vi "Main_Module.vi"(0 "File_hierarchy":string(tree), 11 "Error_In":errorcluster) -> (15 "Error_Out":errorcluster)   [LabVIEW 2023]
uses:
  Controls/Queue_Operation_Select.ctl
  Controls/State_and_Data.ctl
  Controls/Main_Module_Data.ctl
  Classes/Calculator/Calculator.lvclass
  Controls/Object_Data.ctl
  Controls/INI_Operation_Select.ctl
  <vilib>/Utility/miscctls.llb/LVMapReplaceAction.ctl
  Controls/Object_and_instance.ctl
  Drivers/QD_Main.vi
  Drivers/QD_Calci.vi
panel:
  in  "Load":bool
  in  "Save":bool
  in  "Delete":bool
  in  "Add":bool
  in  "Math_Functions":T1(ring) caption="Math Functions"
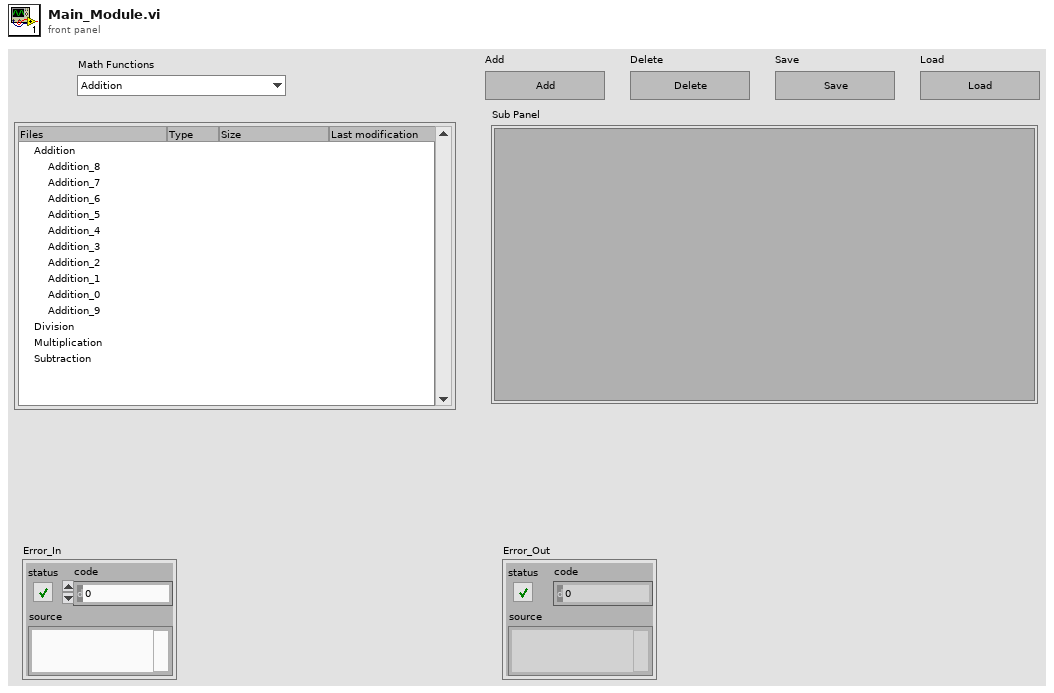
[diagram p1: front panel]
types:
  T1 = enum32{"Addition", "Division", "Multiplication", "Subtraction"}
  T2 = typedef "Queue_Operation_Select.ctl" = enum16{"Obtain_Queue", "Enqueue", "Enqueue_First", "Enqueue_N", "Lossy_Enqueue", "Preview", "Queue_Status", "Dequeue", "Flush", "Release_Queue"}
  T3 = typedef "Main_Module_Data.ctl" = cluster{"File_hierarchy_Reference":refnum<vi>, "Math_Function_Selected":string, "State_and_Data":T4, "Math_Functions":enum16{"Addition", "Division", "Multiplication", "Subtraction"}, "Parent_Class_Path":path, "Calculator.lvclass":refnum<class "Calculator.lvclass">, "Object_Data":T5, "Selected_Tag":string, "Calculator_File_Path":path, "Loaded_VI_Reference":refnum<vi>, "Loaded_Math_Function":string, "Loaded_Tag":string, "Total_Clasees":string[], "INI_File_Path":path}
  T4 = typedef "State_and_Data.ctl" = cluster{"State":string, "Data":variant}
  T5 = typedef "Object_Data.ctl" = map{string, map{string, refnum<class "Calculator.lvclass">}}
  T6 = enum16{"Addition", "Division", "Multiplication", "Subtraction"}
  T7 = typedef "LVMapReplaceAction.ctl" = enum32{"Modify Entry only if found", "Add or Modify Entry", "Delete Entry"}
  T8 = typedef "Object_and_instance.ctl" = cluster{"Object":refnum<class "Calculator.lvclass">, "Insatnce":string}
  T9 = typedef "INI_Operation_Select.ctl" = enum16{"Initialize", "Read", "Read_Key", "Write"}
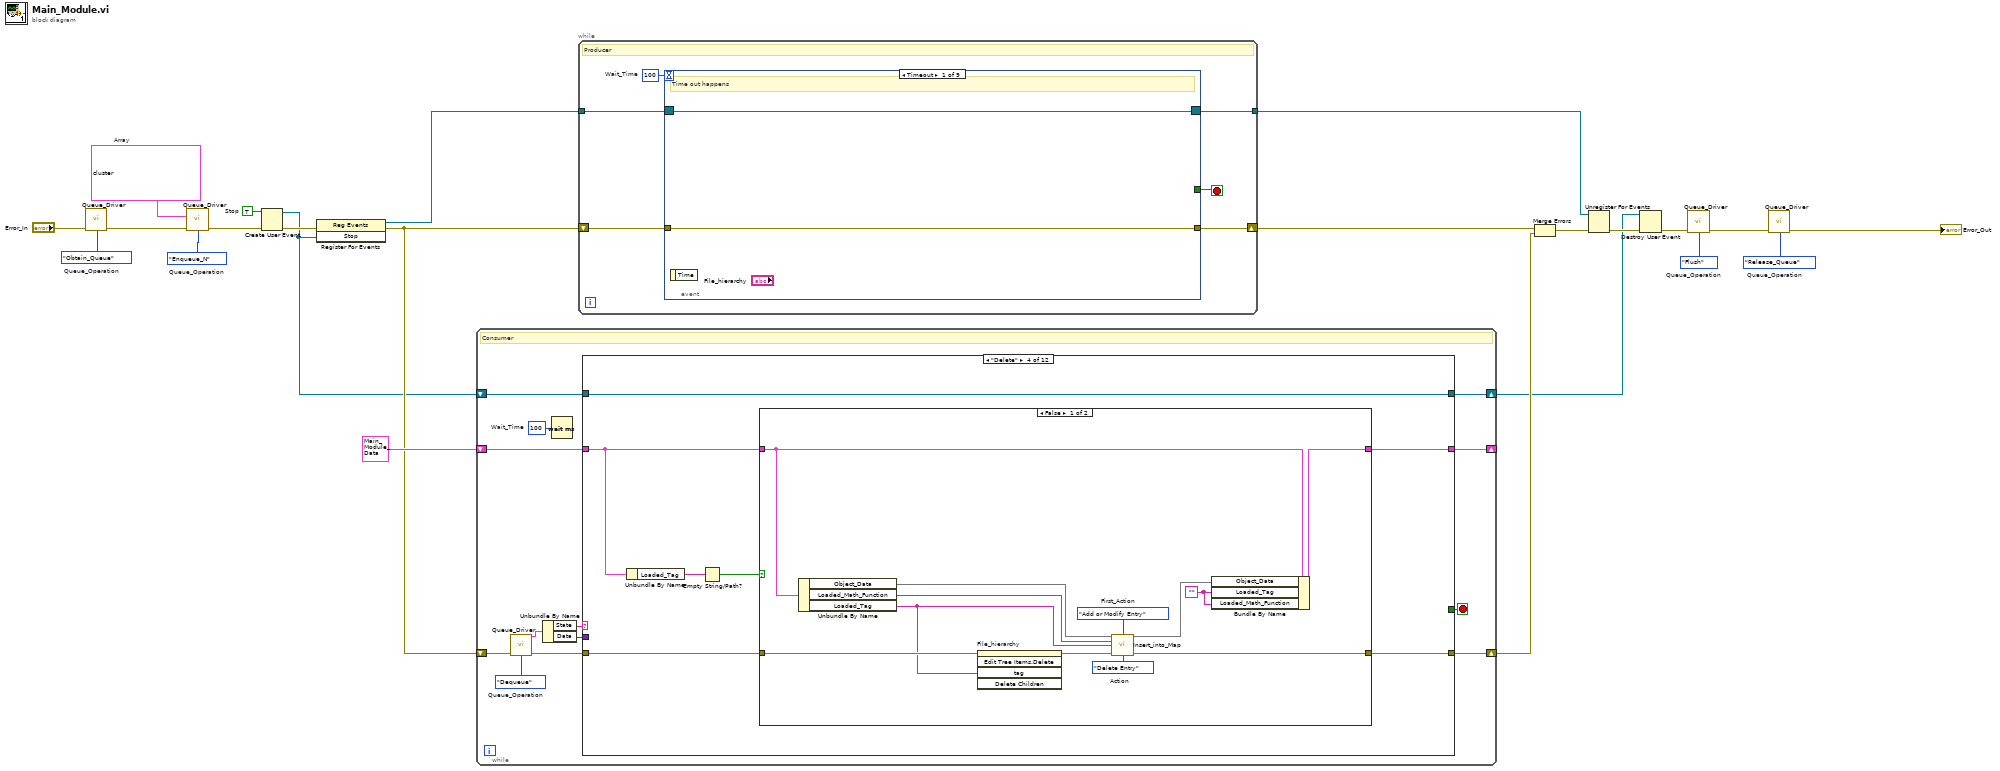
[diagram p0: block diagram]
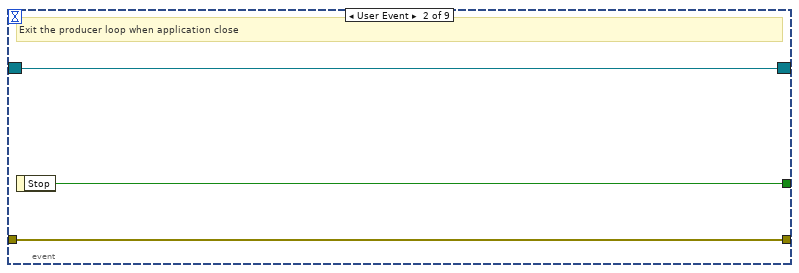
[diagram p2: hidden frame]
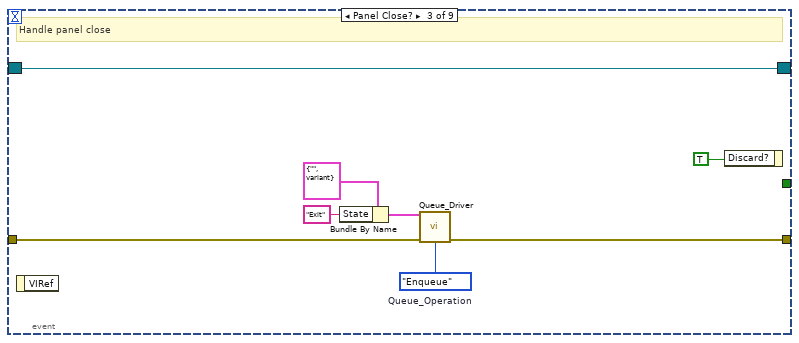
[diagram p3: hidden frame]
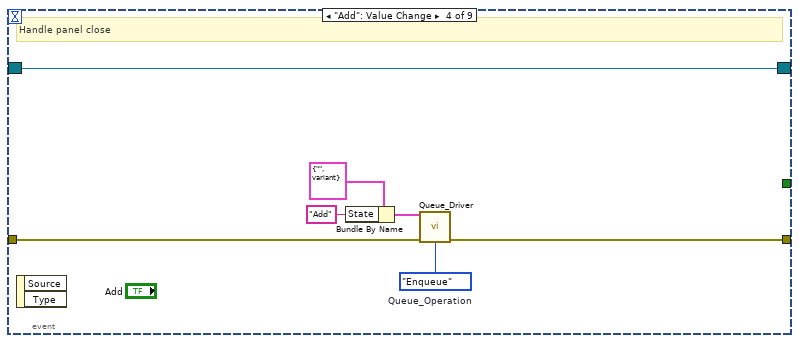
[diagram p4: hidden frame]
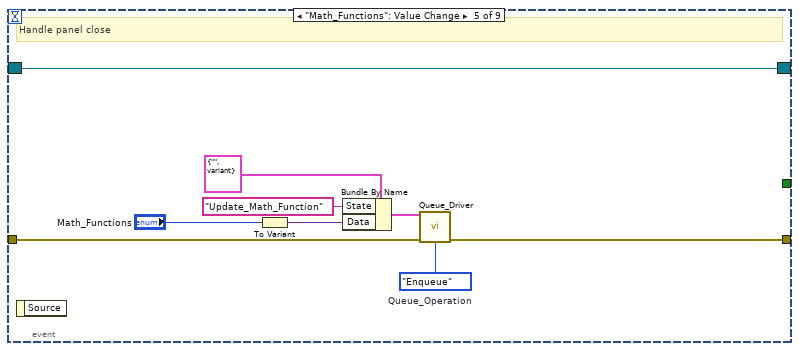
[diagram p5: hidden frame]
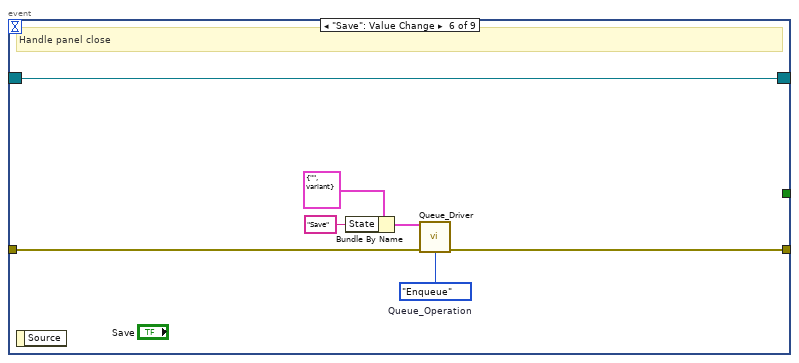
[diagram p6: hidden frame]
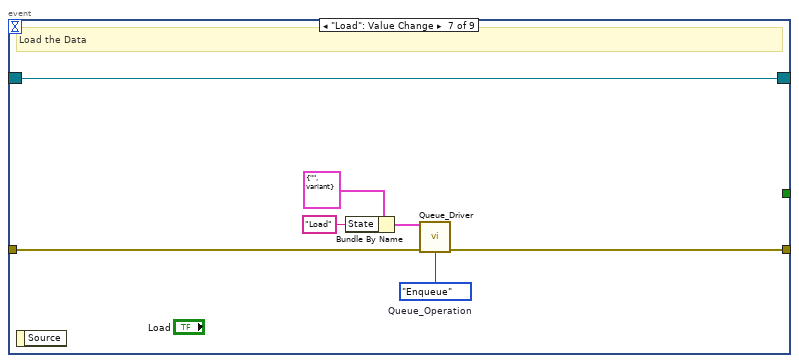
[diagram p7: hidden frame]
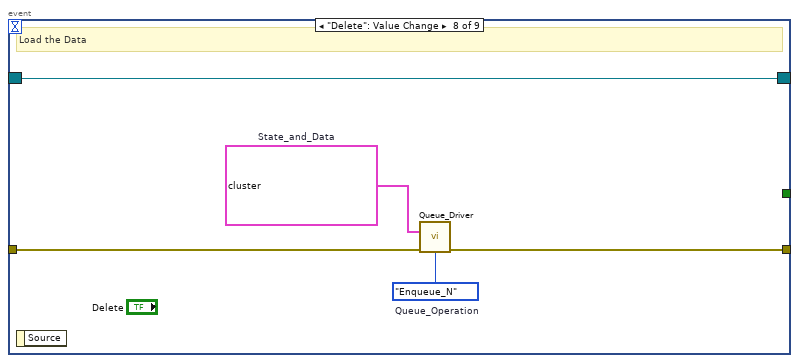
[diagram p8: hidden frame]
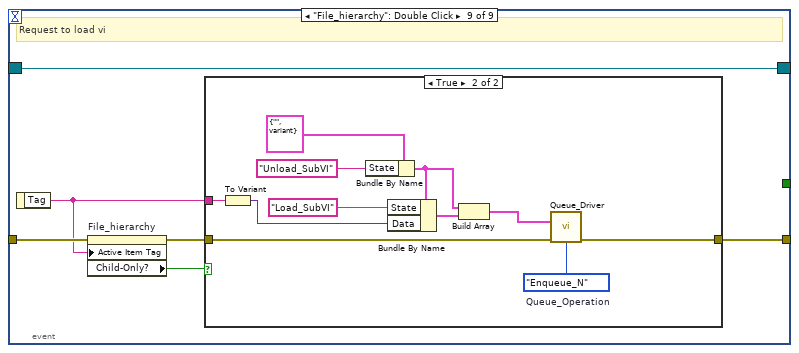
[diagram p9: hidden frame]
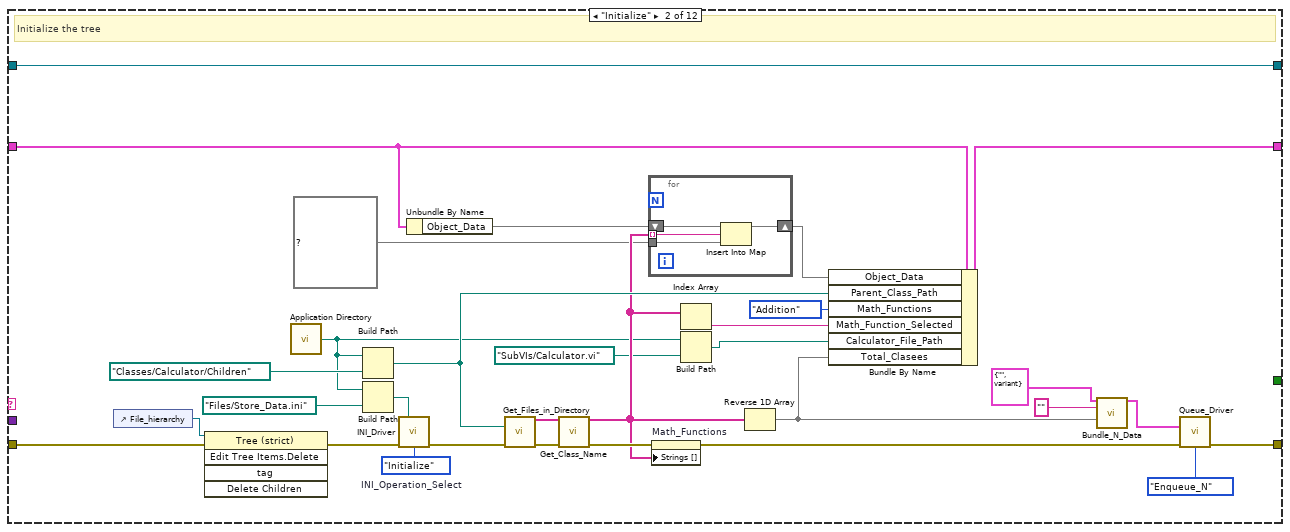
[diagram p12: hidden frame]
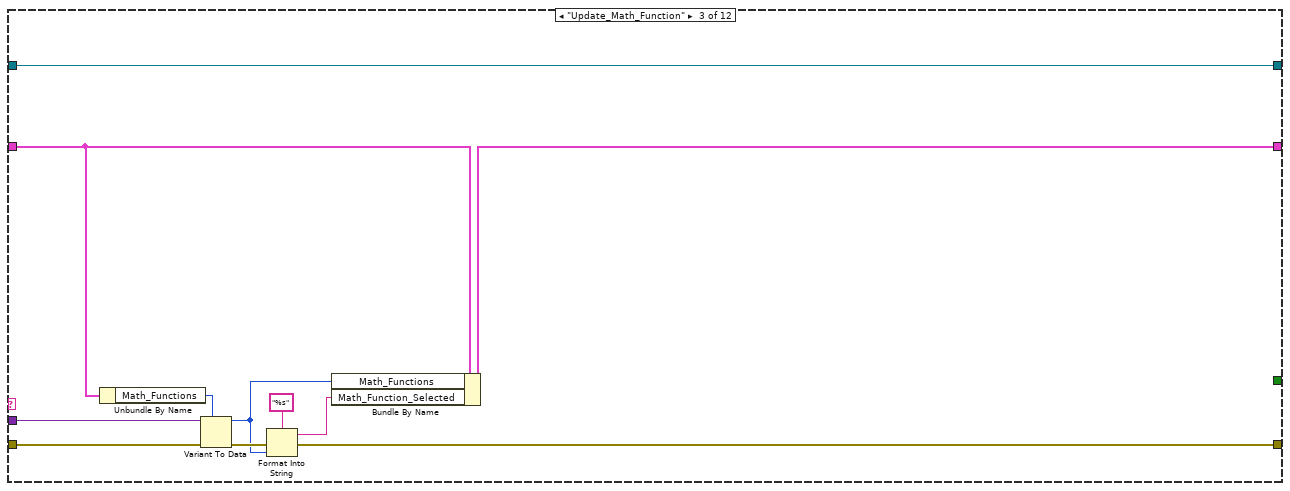
[diagram p13: hidden frame]
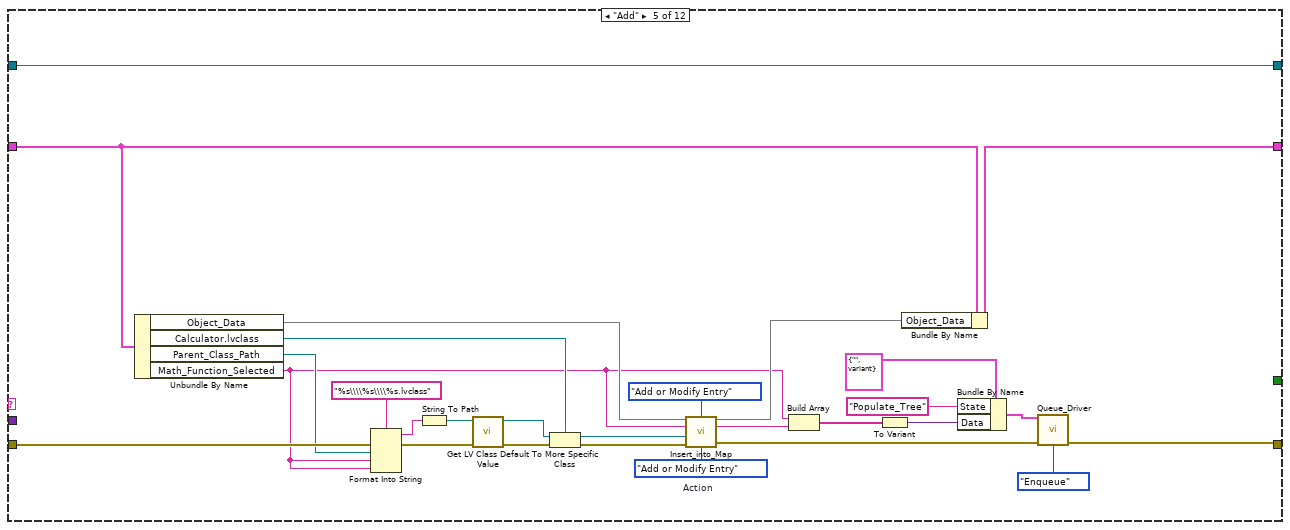
[diagram p15: hidden frame]
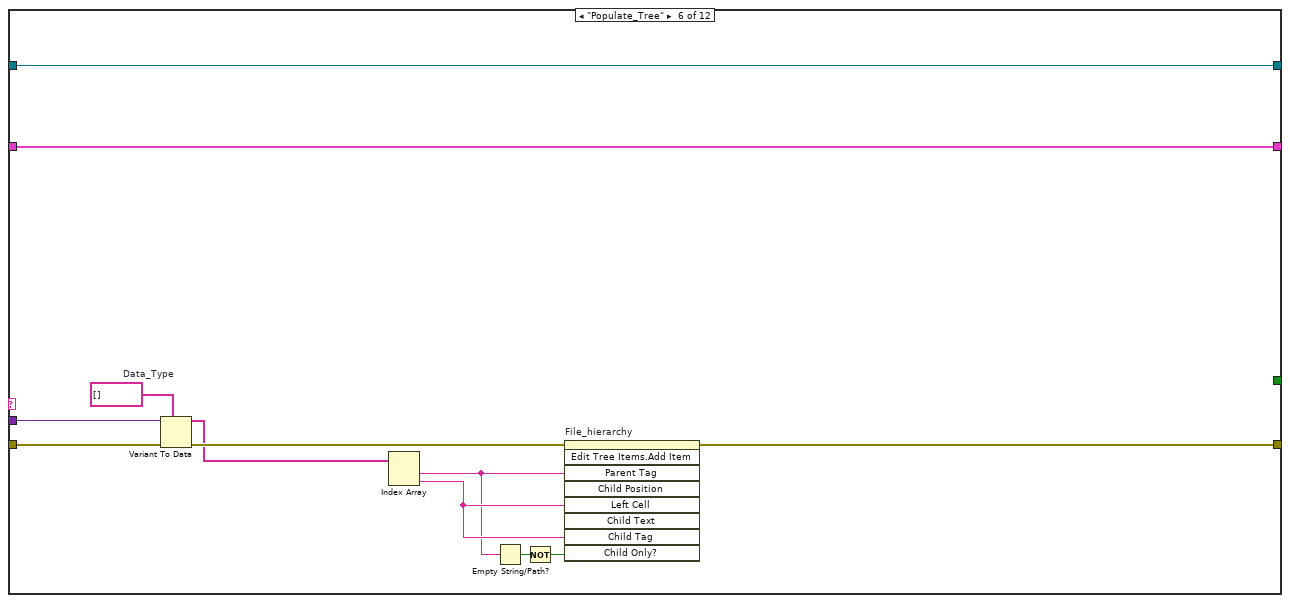
[diagram p16: hidden frame]
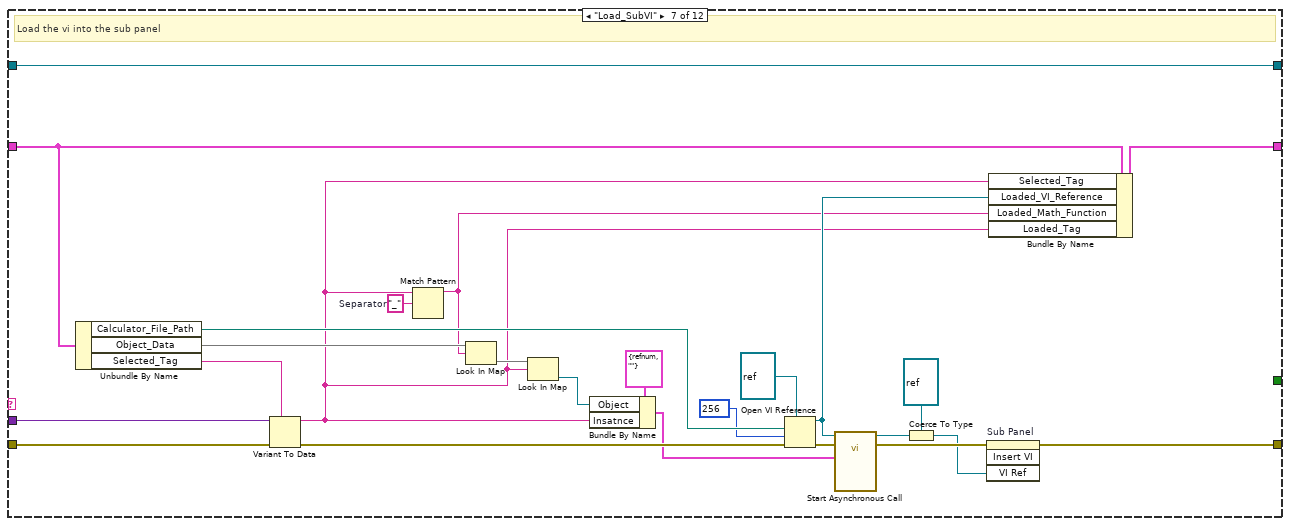
[diagram p17: hidden frame]
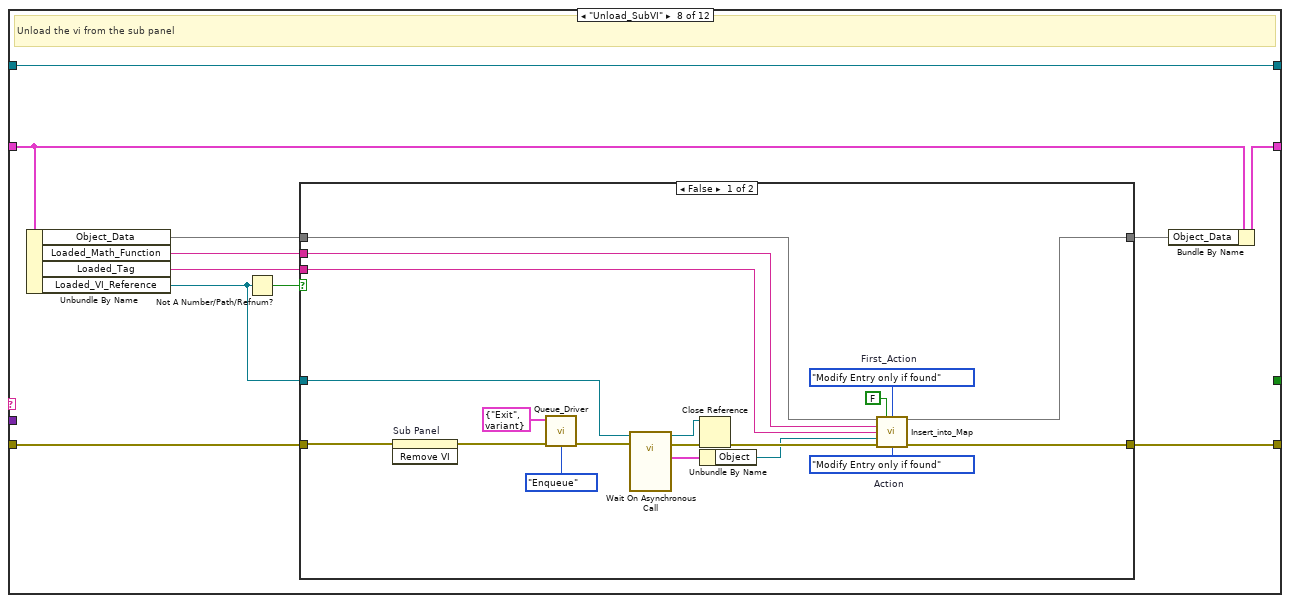
[diagram p18: hidden frame]
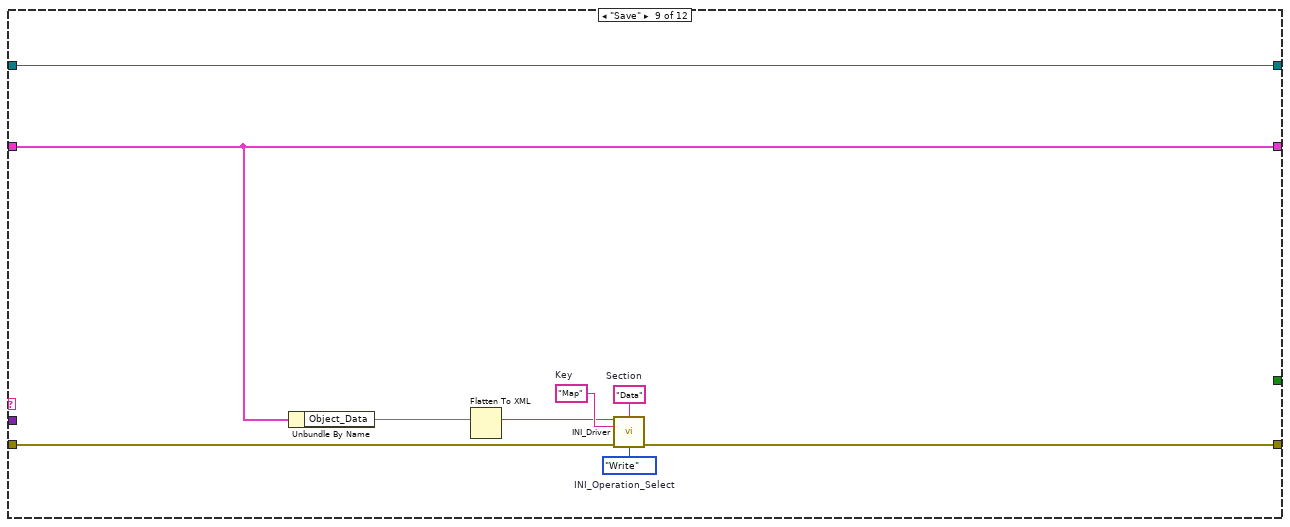
[diagram p20: hidden frame]
diagram:
  w4 = Queue_Operation_Select."Release_Queue"  # Queue_Operation
  w5 = Queue_Operation_Select."Flush"  # Queue_Operation
  w17 = TRUE  # Stop
  w1 = T4[] [{"State"="Initialize", "Data"=variant}, {"State"="Load", "Data"=variant}]  # Array
  w20 = Queue_Operation_Select."Enqueue_N"  # Queue_Operation
  w21 = Queue_Operation_Select."Obtain_Queue"  # Queue_Operation
  n1 = call-poly "Queue_Driver.vi"("Error_In"="Error_In", "Queue_Operation"=w21) -> ("Error_Out"=w22:errorcluster)  [unwired: 11 in, 2 out]
  n2 = call-poly "Queue_Driver.vi"("State_and_Data_N_In"=w1, "Error_In"=w22, "Queue_Operation"=w20) -> ("Error_Out"=w3:errorcluster)  [unwired: 10 in, 2 out]
  n3 = Create User Event(user event datatype=w17, error in=w3) -> (user event=w9:refnum<user-event>, error out=w18:errorcluster)
  n4 = register-events(error in=w18, w9) -> (reference out=w15:refnum<event-registration>, error out=w16:errorcluster)  [unwired: 1 in]
  n5 = while {
    shift-right: [w28] -> w8
    shift-left: w9 -> [w29]
    shift-right: [w27] -> _
    shift-left: T3 {"File_hierarchy_Reference"=refnum, "Math_Function_Selected"="", "State_and_Data"={"State"="", "Data"=variant}, "Math_Functions"=enum."Addition", "Parent_Class_Path"=path "", "Calculator.lvclass"=refnum, "Object_Data"={}, "Selected_Tag"="", "Calculator_File_Path"=path "", "Loaded_VI_Reference"=refnum, "Loaded_Math_Function"="", "Loaded_Tag"="", "Total_Clasees"=[], "INI_File_Path"=path ""} -> [w30]
    shift-right: [w26] -> w13
    shift-left: w16 -> [w36]
    stop <- w25 stop-if-true
    w24 = u32 100  # Wait_Time
    w34 = Queue_Operation_Select."Dequeue"  # Queue_Operation
    # "Consumer"
    n6 = call-poly "Queue_Driver.vi"("Error_In"=w36, "Queue_Operation"=w34) -> ("State_and_Data_Out"=w33:T4, "Error_Out"=w35:errorcluster)  [unwired: 11 in, 1 out]
    n7 = Unbundle By Name(w33) -> ("State"=w32:string, "Data"=w31:variant)
    n8 = Wait (ms)(milliseconds to wait=w24) -> ()  [unwired: 1 out]
    n9 = case shown="\"Delete\"" w32 {
      tunnel: [w39 w61 w78 w90 w116 w143 w169 w179 w210 w213 w248 w258] -> w26
      tunnel: w35 -> [w39 w70 w85 w92 w134 w146 w171 w174 w211 w226 w252 w260]
      tunnel: w31 -> [_ _ w82 _ _ w141 w170 _ _ _ w253 _]
      tunnel: w30 -> [w38 w49 w80 w88 w132 w145 w166 w181 w206 w219 w249 w259]
      tunnel: [w38 w56 w79 w89 w123 w145 w165 w180 w206 w216 w249 w259] -> w27
      tunnel: w29 -> [w37 w69 w84 w91 w133 w144 w167 w182 w212 w227 w254 w257]
      tunnel: [w37 w69 w84 w91 w133 w144 w167 w182 w212 w227 w254 w256] -> w28
      tunnel: [_ _ _ _ _ _ _ _ _ _ _ w255] -> w25
      frame Default {
      }
      frame "Initialize" {
        w42 = INI_Operation_Select."Initialize"  # INI_Operation_Select
        # "Initialize the tree"
        n10 = control-ref of="File_hierarchy"() -> (w68:refnum<vi>)
        n11 = invoke class="Tree (strict)" method="Edit Tree Items.Delete"(reference=w68, error in=w70) -> (error out=w66:errorcluster)  [unwired: 3 in, 4 out]
        n12 = call <vilib>:"Application Directory.vi"() -> ("Application Directory"=w40:path)
        n13 = Build Path(base path=w40, name or relative path=path "Classes/Calculator/Children") -> (appended path=w55:path)
        n14 = Build Path(base path=w40, name or relative path=path "Files/Store_Data.ini") -> (appended path=w41:path)
        n15 = call "INI_Driver.vi"("Config_File_Path"=w41, "Error_Out"=w66, "INI_Operation_Select"=w42) -> ("Error_Out"=w43:errorcluster)  [unwired: 10 in, 2 out]
        n16 = Unbundle By Name(w49) -> ("Object_Data"=w48:T5)
        n17 = call "Get_Files_in_Directory.vi"("File_Path"=w55, "Error_In"=w43) -> ("File_Names_Out"=w63:string[], "Error_Out"=w65:errorcluster)  [unwired: 12 in]
        n18 = call "Get_Class_Name.vi"("File_Names"=w63, "Error_In"=w65) -> ("Class_Names"=w52:string[], "Error_Out"=w64:errorcluster)  [unwired: 12 in]
        n19 = for {
          tunnel: w52 -> [w74] mode=indexing
          tunnel: map{string, refnum<class "Calculator.lvclass">} {} ("Object_Data") -> [w73]
          shift-right: [w72] -> w50
          shift-left: w48 -> [w71]
          n20 = Insert Into Map(map in=w71, key=w74, value=w73) -> (map out=w72:T5)  [unwired: 2 out]
        }
        n21 = property on="Math_Functions" class="Enum (strict)"(error in=w64, "Strings []"=w52) -> (error out=w62:errorcluster)  [unwired: 1 in, 1 out]
        n22 = Index Array(array=w52) -> (element=w53:string)  [unwired: 1 in]
        n23 = Build Path(base path=w40, name or relative path=path "SubVIs/Calculator.vi") -> (appended path=w46:path)
        n24 = Reverse 1D Array(array=w52) -> (reversed array=w45:string[])
        n25 = Bundle By Name(cluster=w49, "Object_Data"=w50, "Parent_Class_Path"=w55, "Math_Functions"=T6."Addition", "Math_Function_Selected"=w53, "Calculator_File_Path"=w46, "Total_Clasees"=w45) -> (w56:T3)
        n26 = call "Bundle_N_Data.vi"("Data_Type"=T4 {"State"="", "Data"=variant} ("State_and_Data"), "Parent"="", "Children_Names"=w45) -> ("Data_Out"=w58:T4[])  [unwired: 12 in]
        n27 = call-poly "Queue_Driver.vi"("State_and_Data_N_In"=w58, "Error_In"=w62, "Queue_Operation"=Queue_Operation_Select."Enqueue_N") -> ("Error_Out"=w61:errorcluster)  [unwired: 10 in, 2 out]
      }
      frame "Update_Math_Function" {
        n28 = Unbundle By Name(w80) -> ("Math_Functions"=w81:T6)
        n29 = Variant To Data(error in=w85, type=w81, Variant=w82) -> (data=w75:T6, error out=w83:errorcluster)
        n30 = Format Into String(format string="%s", error in=w83, w75) -> (resulting string=w76:string, error out=w78:errorcluster)  [unwired: 1 in]
        n31 = Bundle By Name(cluster=w80, "Math_Functions"=w75, "Math_Function_Selected"=w76) -> (w79:T3)
      }
      frame "Delete" {
        n32 = Unbundle By Name(w88) -> ("Loaded_Tag"=w87:string)
        n33 = Empty String/Path?(string/path=w87) -> (empty?=w86:bool)
        n34 = case shown="False" w86 {
          tunnel: w92 -> [w104 w106]
          tunnel: w88 -> [w103 w105]
          tunnel: [w101 w106] -> w90
          tunnel: [w97 w105] -> w89
          frame False {
            w93 = LVMapReplaceAction."Add or Modify Entry"  # First_Action
            w95 = ""
            w94 = LVMapReplaceAction."Delete Entry"  # Action
            n35 = Unbundle By Name(w103) -> ("Object_Data"=w100:T5, "Loaded_Math_Function"=w99:string, "Loaded_Tag"=w98:string)
            n36 = invoke on="File_hierarchy" class="Tree (strict)" method="Edit Tree Items.Delete"(error in=w104, "tag"=w98) -> (error out=w102:errorcluster)  [unwired: 3 in, 4 out]
            n37 = call "Insert_into_Map.vi"("Object_Data_In"=w100, "First_Action"=w93, "First_Key"=w99, "Second_Key"=w98, "Error_In"=w102, "Second_Action"=w94) -> ("Object_Data_Out"=w96:T5, "error out"=w101:errorcluster)  [unwired: 7 in, 1 out]
            n38 = Bundle By Name(cluster=w103, "Object_Data"=w96, "Loaded_Tag"=w95, "Loaded_Math_Function"=w95) -> (w97:T3)
          }
          frame True {
          }
        }
      }
      frame "Add" {
        w110 = LVMapReplaceAction."Add or Modify Entry"  # Action
        n39 = Unbundle By Name(w132) -> ("Object_Data"=w122:T5, "Calculator.lvclass"=w125:refnum<class "Calculator.lvclass">, "Parent_Class_Path"=w130:path, "Math_Function_Selected"=w111:string)
        n40 = Format Into String(format string="%s\\\\%s\\\\%s.lvclass", error in=w134, w130, w111, w111) -> (resulting string=w129:string, error out=w128:errorcluster)  [unwired: 1 in]
        n41 = String To Path(string=w129) -> (path=w127:path)
        n42 = call <vilib>:"Get LV Class Default Value.vi"("error in (no error)"=w128, "class path"=w127) -> ("error out"=w124:errorcluster, "object"=w126:refnum<class>)  [unwired: 8 in]
        n43 = To More Specific Class(target class=w125, reference=w126, error in=w124) -> (specific class reference=w108:refnum<class "Calculator.lvclass">, error out=w109:errorcluster)
        n44 = call "Insert_into_Map.vi"("Object_Data_In"=w122, "First_Action"=LVMapReplaceAction."Add or Modify Entry", "First_Key"=w111, "Calculator.lvclass"=w108, "Error_In"=w109, "Second_Action"=w110) -> ("Object_Data_Out"=w121:T5, "Second_Key"=w115:string, "error out"=w117:errorcluster)  [unwired: 7 in]
        n45 = Build Array(w111, w115) -> (w112:string[])
        n46 = To Variant(anything=w112) -> (Variant=w113:variant)
        n47 = Bundle By Name(cluster=w132, "Object_Data"=w121) -> (w123:T3)
        n48 = Bundle By Name(cluster=T4 {"State"="", "Data"=variant} ("State_and_Data_In"), "State"="Populate_Tree", "Data"=w113) -> (w120:T4)
        n49 = call-poly "Queue_Driver.vi"("State_and_Data_In"=w120, "Error_In"=w117, "Queue_Operation"=Queue_Operation_Select."Enqueue") -> ("Error_Out"=w116:errorcluster)  [unwired: 10 in, 2 out]
      }
      frame "Populate_Tree" {
        w140 = string[] []  # Data_Type
        n50 = Variant To Data(error in=w146, type=w140, Variant=w141) -> (data=w139:string[], error out=w142:errorcluster)
        n51 = Index Array(array=w139) -> (element #1=w137:string, element #2=w138:string)  [unwired: 2 in]
        n52 = Empty String/Path?(string/path=w137) -> (empty?=w136:bool)
        n53 = Not(x=w136) -> (.not. x?=w135:bool)
        n54 = invoke on="File_hierarchy" class="Tree (strict)" method="Edit Tree Items.Add Item"(error in=w142, "Parent Tag"=w137, "Left Cell"=w138, "Child Tag"=w138, "Child Only?"=w135) -> (error out=w143:errorcluster)  [unwired: 4 in, 8 out]
      }
      frame "Load_SubVI" {
        w152 = "_"  # Separator
        # "Load the vi into the sub panel"
        n55 = Unbundle By Name(w166) -> ("Calculator_File_Path"=w159:path, "Object_Data"=w161:T5, "Selected_Tag"=w168:string)
        n56 = Variant To Data(error in=w171, type=w168, Variant=w170) -> (data=w147:string, error out=w153:errorcluster)
        n57 = Match Pattern(string=w147, regular expression=w152) -> (before substring=w151:string)  [unwired: 1 in, 3 out]
        n58 = Look In Map(map=w161, key=w151) -> (value=w160:map{string, refnum<class "Calculator.lvclass">})  [unwired: 1 in, 1 out]
        n59 = Look In Map(map=w160, key=w147) -> (value=w148:refnum<class "Calculator.lvclass">)  [unwired: 1 in, 1 out]
        n60 = Bundle By Name(cluster=T8 {"Object"=refnum, "Insatnce"=""}, "Object"=w148, "Insatnce"=w147) -> (w149:T8)
        n61 = Open VI Reference(type specifier VI Refnum (for type only)=refnum<vi> refnum, vi path=w159, options=256, error in (no error)=w153) -> (vi reference=w154:refnum<vi>, error out=w164:errorcluster)  [unwired: 2 in]
        n62 = call-by-ref "Start Asynchronous Call"(reference=w154, error in=w164, "Object_and_Instance_In"=w149) -> (reference out=w158:refnum<vi>, error out=w163:errorcluster)  [unwired: 12 in, 3 out]
        n63 = Coerce To Type(0:w158, 1:refnum<vi> refnum ("This VI")) -> (2:w155:refnum<vi>)
        n64 = invoke on="Sub Panel" class="SubPnl" method="Insert VI"(error in=w163, "VI Ref"=w155) -> (error out=w169:errorcluster)  [unwired: 2 in, 3 out]
        n65 = Bundle By Name(cluster=w166, "Selected_Tag"=w147, "Loaded_VI_Reference"=w154, "Loaded_Math_Function"=w151, "Loaded_Tag"=w147) -> (w165:T3)
      }
      frame "Unload_SubVI" {
        # "Unload the vi from the sub panel"
        n66 = Unbundle By Name(w181) -> ("Object_Data"=w178:T5, "Loaded_Math_Function"=w177:string, "Loaded_Tag"=w176:string, "Loaded_VI_Reference"=w173:refnum<vi>)
        n67 = Not A Number/Path/Refnum?(number/path/refnum=w173) -> (NaN/Path/Refnum?=w172:bool)
        n68 = case shown="False" w172 {
          tunnel: w174 -> [w192 w202]
          tunnel: w173 -> [w200 _]
          tunnel: [w198 w202] -> w179
          tunnel: w178 -> [w197 w203]
          tunnel: w177 -> [w196 _]
          tunnel: w176 -> [w195 _]
          tunnel: [w193 w203] -> w175
          frame False {
            w183 = LVMapReplaceAction."Modify Entry only if found"  # First_Action
            w194 = LVMapReplaceAction."Modify Entry only if found"  # Action
            n69 = invoke on="Sub Panel" class="SubPnl" method="Remove VI"(error in=w192) -> (error out=w185:errorcluster)  [unwired: 2 in, 2 out]
            n70 = call-poly "Queue_Driver.vi"("State_and_Data_In"=T4 {"State"="Exit", "Data"=variant} ("State_and_Data"), "Error_In"=w185, "Queue_Operation"=Queue_Operation_Select."Enqueue") -> ("Error_Out"=w191:errorcluster)  [unwired: 10 in, 2 out]
            n71 = call-by-ref "Wait On Asynchronous Call"(reference=w200, error in=w191) -> (reference out=w199:refnum<vi>, error out=w201:errorcluster, "Object_and_instance_Out"=w187:T8)  [unwired: 13 in, 2 out]
            n72 = Close Reference(reference=w199, error in (no error)=w201) -> (error out=w188:errorcluster)
            n73 = Unbundle By Name(w187) -> ("Object"=w186:refnum<class "Calculator.lvclass">)
            n74 = call "Insert_into_Map.vi"("Object_Data_In"=w197, "Create_Second_Key (T)"=FALSE, "First_Action"=w183, "First_Key"=w196, "Second_Key"=w195, "Calculator.lvclass"=w186, "Error_In"=w188, "Second_Action"=w194) -> ("Object_Data_Out"=w193:T5, "error out"=w198:errorcluster)  [unwired: 5 in, 1 out]
          }
          frame True {
          }
        }
        n75 = Bundle By Name(cluster=w181, "Object_Data"=w175) -> (w180:T3)
      }
      frame "Save" {
        w207 = "Map"  # Key
        w208 = "Data"  # Section
        w209 = INI_Operation_Select."Write"  # INI_Operation_Select
        n76 = Unbundle By Name(w206) -> ("Object_Data"=w205:T5)
        n77 = Flatten To XML(6:w205) -> (2:w204:string)
        n78 = call "INI_Driver.vi"("Data_In"=w204, "Section"=w208, "Key"=w207, "Error_Out"=w211, "INI_Operation_Select"=w209) -> ("Error_Out"=w210:errorcluster)  [unwired: 8 in, 2 out]
      }
      frame "Load" {
        w222 = "Map"  # Key
        w223 = "Data"  # Section
        w224 = INI_Operation_Select."Read"  # INI_Operation_Select
        n79 = call "INI_Driver.vi"("Section"=w223, "Key"=w222, "Error_Out"=w226, "INI_Operation_Select"=w224) -> ("Data_Out"=w220:string, "Error_Out"=w225:errorcluster)  [unwired: 9 in, 1 out]
        n80 = Unbundle By Name(w219) -> ("Total_Clasees"=w214:string[], "Object_Data"=w218:T5)
        n81 = Unflatten From XML(xml string=w220, type=w218, error in (no error)=w225) -> (value=w215:T5, error out=w221:errorcluster)
        n82 = Bundle By Name(cluster=w219, "Object_Data"=w215) -> (w216:T3)
        n83 = for {
          tunnel: w215 -> [w231]
          tunnel: w214 -> [w229] mode=indexing
          tunnel: w221 -> [w233]
          tunnel: [w228] -> w217 mode=indexing
          n84 = Look In Map(map=w231, key=w229) -> (value=w230:map{string, refnum<class "Calculator.lvclass">})  [unwired: 1 in, 1 out]
          n85 = for {
            tunnel: w230 -> [w241] mode=indexing
            tunnel: w229 -> [w235]
            tunnel: w233 -> [w244]
            tunnel: [w243] -> w232 mode=indexing
            w242 = Queue_Operation_Select."Enqueue"  # Queue_Operation
            n86 = Unbundle(w241) -> (w234:string)  [unwired: 1 out]
            n87 = Build Array(w235, w234) -> (w236:string[])
            n88 = To Variant(anything=w236) -> (Variant=w238:variant)
            n89 = Bundle By Name(cluster=T4 {"State"="", "Data"=variant} ("State_and_Data"), "State"="Populate_Tree", "Data"=w238) -> (w239:T4)
            n90 = call-poly "Queue_Driver.vi"("State_and_Data_In"=w239, "Error_In"=w244, "Queue_Operation"=w242) -> ("Error_Out"=w243:errorcluster)  [unwired: 10 in, 2 out]
          }
          n91 = Merge Errors(w232) -> (w228:errorcluster)
        }
        n92 = Merge Errors(w217) -> (w213:errorcluster)
      }
      frame "Error" {
        w247 = Queue_Operation_Select."Enqueue"  # Queue_Operation
        # "Handle error"
        n93 = Variant To Data(error in=w252, type=w252, Variant=w253) -> (data=w246:errorcluster, error out=w251:errorcluster)
        n94 = call "Analyse_Error.vi"("Error_Under_Analysis"=w246, "Error_In"=w251) -> ("State_and_Data"=w245:T4, "Error_Out"=w250:errorcluster)  [unwired: 12 in]
        n95 = call-poly "Queue_Driver.vi"("State_and_Data_In"=w245, "Error_In"=w250, "Queue_Operation"=w247) -> ("Error_Out"=w248:errorcluster)  [unwired: 10 in, 2 out]
      }
      frame "Exit" {
        # "Exit the application"
        n96 = disable-structure shown="RUN_TIME_ENGINE==True" {
          disable-tunnel: [w261 w265] -> w255
          frame condition #0 {
            w261 = TRUE  # Stop
            # "Run time mode"
          }
          frame condition #1 (active) {
            w262 = "No"  # Cont
            w263 = "Yes"  # Stop
            w264 = "Do you want to stop execution"  # Message
            # "Developer mode"
            n97 = Two Button Dialog(message=w264, 1:w262, 2:w263) -> (T button?=w265:bool)
          }
        }
        n98 = Generate User Event(user event=w257, event data cluster=w255, error in=w260) -> (user event out=w256:refnum<user-event>, error out=w258:errorcluster)  [unwired: 1 in]
      }
    }
  }
  n99 = while {
    tunnel: w15 -> [w270]
    shift-right: [w268] -> w14
    shift-left: w16 -> [w271]
    tunnel: [w266] -> w11
    stop <- w269 stop-if-true
    w267 = 100  # Wait_Time
    # "Producer"
    n100 = event shown="[0] Timeout" {
      selector: w270 -> [w272 w274 w277 w285 w294 w301 w308 w316 w320]
      dyn-events: [w272 w274 w277 w285 w294 w301 w308 w316 w320] -> w266
      timeout: w267 -> [_ _ _ _ _ _ _ _ _]
      tunnel: w271 -> [w273 w276 w281 w289 w298 w305 w312 w318 w324]
      tunnel: [w273 w276 w280 w288 w297 w304 w311 w317 w325] -> w268
      tunnel: [_ w275 _ _ _ _ _ _ _] -> w269
      event Timeout {
        # "Time out happens"
        n101 = event-data() -> ()  [unwired: 1 in, 1 out]
      }
      event User Event {
        # "Exit the producer loop when application close"
        n102 = event-data() -> ("Stop"=w275:bool)  [unwired: 1 in]
      }
      event Panel Close? {
        w282 = Queue_Operation_Select."Enqueue"  # Queue_Operation
        # "Handle panel close"
        n103 = event-data() -> ()  [unwired: 1 in, 1 out]
        n104 = Bundle By Name(cluster=T4 {"State"="", "Data"=variant} ("State_and_Data"), "State"="Exit") -> (w279:T4)
        n105 = call-poly "Queue_Driver.vi"("State_and_Data_In"=w279, "Error_In"=w281, "Queue_Operation"=w282) -> ("Error_Out"=w280:errorcluster)  [unwired: 10 in, 2 out]
        n106 = event-data("Discard?"=TRUE) -> ()  [unwired: 1 in, 1 out]
      }
      event "Add": Value Change {
        w290 = Queue_Operation_Select."Enqueue"  # Queue_Operation
        # "Handle panel close"
        n107 = event-data() -> ()  [unwired: 1 in, 2 out]
        n108 = Bundle By Name(cluster=T4 {"State"="", "Data"=variant} ("State_and_Data"), "State"="Add") -> (w287:T4)
        n109 = call-poly "Queue_Driver.vi"("State_and_Data_In"=w287, "Error_In"=w289, "Queue_Operation"=w290) -> ("Error_Out"=w288:errorcluster)  [unwired: 10 in, 2 out]
      }
      event "Math_Functions": Value Change {
        w299 = Queue_Operation_Select."Enqueue"  # Queue_Operation
        # "Handle panel close"
        n110 = event-data() -> ()  [unwired: 1 in, 1 out]
        n111 = To Variant(anything="Math_Functions") -> (Variant=w292:variant)
        n112 = Bundle By Name(cluster=T4 {"State"="", "Data"=variant} ("State_and_Data"), "State"="Update_Math_Function", "Data"=w292) -> (w296:T4)
        n113 = call-poly "Queue_Driver.vi"("State_and_Data_In"=w296, "Error_In"=w298, "Queue_Operation"=w299) -> ("Error_Out"=w297:errorcluster)  [unwired: 10 in, 2 out]
      }
      event "Save": Value Change {
        w306 = Queue_Operation_Select."Enqueue"  # Queue_Operation
        # "Handle panel close"
        n114 = event-data() -> ()  [unwired: 1 in, 1 out]
        n115 = Bundle By Name(cluster=T4 {"State"="", "Data"=variant} ("State_and_Data"), "State"="Save") -> (w303:T4)
        n116 = call-poly "Queue_Driver.vi"("State_and_Data_In"=w303, "Error_In"=w305, "Queue_Operation"=w306) -> ("Error_Out"=w304:errorcluster)  [unwired: 10 in, 2 out]
      }
      event "Load": Value Change {
        w313 = Queue_Operation_Select."Enqueue"  # Queue_Operation
        # "Load the Data"
        n117 = event-data() -> ()  [unwired: 1 in, 1 out]
        n118 = Bundle By Name(cluster=T4 {"State"="", "Data"=variant} ("State_and_Data"), "State"="Load") -> (w310:T4)
        n119 = call-poly "Queue_Driver.vi"("State_and_Data_In"=w310, "Error_In"=w312, "Queue_Operation"=w313) -> ("Error_Out"=w311:errorcluster)  [unwired: 10 in, 2 out]
      }
      event "Delete": Value Change {
        w319 = Queue_Operation_Select."Enqueue_N"  # Queue_Operation
        w315 = T4[] [{"State"="Unload_SubVI", "Data"=variant}, {"State"="Delete", "Data"=variant}]  # State_and_Data
        # "Load the Data"
        n120 = event-data() -> ()  [unwired: 1 in, 1 out]
        n121 = call-poly "Queue_Driver.vi"("State_and_Data_N_In"=w315, "Error_In"=w318, "Queue_Operation"=w319) -> ("Error_Out"=w317:errorcluster)  [unwired: 10 in, 2 out]
      }
      event "File_hierarchy": Double Click {
        # "Request to load vi"
        n122 = event-data() -> ("Tag"=w322:string)  [unwired: 1 in]
        n123 = property on="File_hierarchy" class="Tree (strict)"(error in=w324, "Active Item Tag"=w322) -> (error out=w323:errorcluster, "Child-Only?"=w321:bool)  [unwired: 1 in, 1 out]
        n124 = case shown="True" w321 {
          tunnel: [w326 w337] -> w325
          tunnel: w323 -> [w326 w333]
          tunnel: w322 -> [_ w332]
          frame False {
          }
          frame True {
            w334 = Queue_Operation_Select."Enqueue_N"  # Queue_Operation
            n125 = To Variant(anything=w332) -> (Variant=w335:variant)
            n126 = Bundle By Name(cluster=T4 {"State"="", "Data"=variant} ("State_and_Data"), "State"="Unload_SubVI") -> (w329:T4)
            n127 = Bundle By Name(cluster=w329, "State"="Load_SubVI", "Data"=w335) -> (w330:T4)
            n128 = Build Array(w329, w330) -> (w328:T4[])
            n129 = call-poly "Queue_Driver.vi"("State_and_Data_N_In"=w328, "Error_In"=w333, "Queue_Operation"=w334) -> ("Error_Out"=w337:errorcluster)  [unwired: 10 in, 2 out]
          }
        }
      }
    }
  }
  n130 = Merge Errors(w14, w13) -> (w12:errorcluster)
  n131 = Unregister For Events(event registration refnum=w11, error in=w12) -> (error out=w10:errorcluster)
  n132 = Destroy User Event(user event=w8, error in=w10) -> (error out=w7:errorcluster)
  n133 = call-poly "Queue_Driver.vi"("Error_In"=w7, "Queue_Operation"=w5) -> ("Error_Out"=w6:errorcluster)  [unwired: 11 in, 2 out]
  n134 = call-poly "Queue_Driver.vi"("Error_In"=w6, "Queue_Operation"=w4) -> ("Error_Out"=→"Error_Out":errorcluster)  [unwired: 11 in, 2 out]
